vi "Framework Test2.vi"() -> ()   [LabVIEW 2017]
uses:
  Typedefs/DSF Engine Framework Configuration.ctl
  Typedefs/DSF Engine Plugin Configuration.ctl
  Typedefs/DSF Timing Info.ctl
  Typedefs/DSF Engine Plugin Thread Configuration.ctl
  Typedefs/DSF Settings Info.ctl
  Typedefs/DSF Engine Transfer Group Configuration.ctl
  Typedefs/DSF Direction.ctl
  Typedefs/DSF Engine Transfer Configuration.ctl
  Typedefs/DSF Byte Order.ctl
  Typedefs/DSF Engine Channel Configuration.ctl
  Typedefs/DSF Data Type.ctl
  Typedefs/DSF Timeout Behavior.ctl
  Classes/Framework/Framework Options.ctl
  Typedefs/DSF FIFO Options.ctl
  Classes/Thread/Thread Options.ctl
  Typedefs/DSF Plugin Options.ctl
  Typedefs/DSF Performance Options.ctl
  Classes/Framework/Data Server Options.ctl
  <vilib>/NI/Memory Manager/Classes/Pointer/Pointer.lvclass/Pointer.ctl
  <vilib>/NI/Memory Manager/Classes/Pointer/Write Bool.vi
  <vilib>/NI/Memory Manager/Classes/Pointer/Write DBL.vi
  <vilib>/NI/Memory Manager/Classes/Pointer/Read Bool.vi
  <vilib>/NI/Memory Manager/Classes/Pointer/Set Address.vi
  <vilib>/NI/Memory Manager/Classes/Pointer/Set Size.vi
  <vilib>/NI/Memory Manager/Classes/Pointer/Set Internal.vi
  <vilib>/NI/Memory Manager/Classes/Pointer/Write (No Check).vi
  <vilib>/NI/Memory Manager/Classes/Pointer/Write (No Check) Bool.vi
  <vilib>/NI/Memory Manager/Classes/Pointer/Check Move.vi
  <vilib>/NI/Memory Manager/Classes/Pointer/Check Null Pointer.vi
  <vilib>/NI/Memory Manager/Classes/Pointer/Clear (No Check).vi
  <vilib>/NI/Memory Manager/Classes/Pointer/Check Length.vi
  <vilib>/NI/Memory Manager/Classes/Pointer/Write (No Check) DBL.vi
  <vilib>/NI/Memory Manager/Classes/Pointer/Read (No Check).vi
  <vilib>/NI/Memory Manager/Classes/Pointer/Read (No Check) Bool.vi
  <vilib>/NI/Memory Manager/Classes/Pointer/Get Internal.vi
  <vilib>/NI/Memory Manager/Classes/Pointer/Errors.vi
  <vilib>/NI/Memory Manager/Classes/Pointer/Zone.vi
  <vilib>/NI/Memory Manager/Classes/Pointer/Check Count.vi
  <vilib>/NI/Memory Manager/Classes/Pointer/Check Bounds (Power of 2).vi
  <vilib>/NI/Memory Manager/Classes/Pointer/Null Pointer.vi
  <vilib>/NI/Memory Manager/Classes/Pointer/Is Null.vi
  <vilib>/NI/Memory Manager/Classes/Pointer/Check Bounds (Pointer).vi
  <vilib>/NI/Memory Manager/Classes/Pointer/Create Error.vi
  <vilib>/NI/Memory Manager/Classes/Pointer/Out of Bounds.vi
  <vilib>/NI/Memory Manager/Classes/Pointer/Check Bounds.vi
  <vilib>/NI/Memory Manager/Constants/Constants.vi
  <vilib>/NI/Memory Manager/Constants/Library Name.vi
  <vilib>/NI/Memory Manager/Classes/Pointer/Pointer Error Info.vi
  <vilib>/NI/Memory Manager/Constants/Pointer Class Name.vi
  <vilib>/NI/Memory Manager/Classes/Pointer/Write Pointer Size to Error.vi
  <vilib>/NI/Memory Manager/Classes/Pointer/Check Bounds (Buffer).vi
  <vilib>/NI/Memory Manager/Classes/Pointer/Buffer Underflow.vi
  <vilib>/NI/Memory Manager/VIs/New Error Cluster.vi
  <vilib>/NI/Memory Manager/VIs/New Error Cluster (512B).vi
  <vilib>/NI/Memory Manager/VIs/Set Error Status.vi
  <vilib>/NI/Memory Manager/VIs/Set Error Code.vi
  <vilib>/NI/Memory Manager/VIs/Set Error Source.vi
  <vilib>/NI/Memory Manager/VIs/Write String to Source.vi
  <vilib>/NI/Memory Manager/VIs/Write Numeric to Source.vi
  <vilib>/NI/Memory Manager/VIs/Write Numeric Scalar to Source (Base10 U64).vi
  <vilib>/NI/Memory Manager/Classes/Pointer/Pointer.lvclass
  Classes/Framework/Framework.lvclass
  Classes/Configuration/Configuration Session.lvclass
  DSF Core.lvlib
  Classes/Thread/Thread.lvclass
panel:
  in  "first channel":dbl
  in  "components directory":path
  in  "dsf configuration file path":path=path "C:/Users/Admin/Desktop/test.dsf"
  out "iteration":u64
  out "error out":errorcluster
  in  "framework options":T1={"FIFO Options"={"Infinite Timeouts"=FALSE}, "Thread Options"={"Show FP On Call"=TRUE, "Close FP After Call"=TRUE, "Allow Debugging"=TRUE}, "Plugin Options"={"Default Components"=TRUE}, "Performance Options"={"Measure Period"=TRUE, "Measure Rx/Tx Duration"=TRUE}, "Data Server Options"={"Enable Data Server"=TRUE, "Period"=50}} {"Data Server Options"."Period" format="%d ms"}
  in  "framework configuration":T7={"Plugins"=[{"name"="UDP", "components"=["UDP"], "cycle timing"={"priority"=100, "decimation"=1, "offset"=0}, "threads"=[{"buffer converter settings"=[], "transceiver settings"=[{"key"="Local Port", "value"="50000"}], "custom settings"=[], "processor"=-2, "priority offset"=0}, {"buffer converter settings"=[], "transceiver settings"=[{"key"="Local Port", "value"="50001"}], "custom settings"=[], "processor"=-2, "priority offset"=0}, {"buffer converter settings"=[], "transceiver settings"=[{"key"="Local Port", "value"="50002"}], "custom settings"=[], "processor"=-2, "priority offset"=0}, {"buffer converter settings"=[], "transceiver settings"=[{"key"="Local Port", "value"="50003"}], "custom settings"=[], "processor"=-2, "priority offset"=0}], "Transfer Groups"=[{"name"="Group0", "direction"=enum."Tx", "cycle timing"={"priority"=100, "decimation"=1, "offset"=0}, "thread index"=0, "settings"=[], "Transfers"=[{"name"="Transfer0", "byte order"=enum."big-endian", "settings"=[{"key"="Destination Port", "value"="60000"}, {"key"="Destination Address", "value"="localhost"}], "channels"=[{"string offset"=0, "string data type"=enum."SGL", "engine data type"=enum."DBL", "name"="Temp", "settings"=[], "units"="V"}, {"string offset"=4, "string data type"=enum."DBL", "engine data type"=enum."DBL", "name"="RPM", "settings"=[], "units"="V"}, {"string offset"=12, "string data type"=enum."Bool", "engine data type"=enum."DBL", "name"="LED", "settings"=[], "units"="V"}, {"string offset"=792, "string data type"=enum."U64", "engine data type"=enum."DBL", "name"="Count", "settings"=[], "units"="V"}]}], "timeout behavior"=enum."Increment Late Count"}], "settings"=[]}]}
  in  "stop":bool
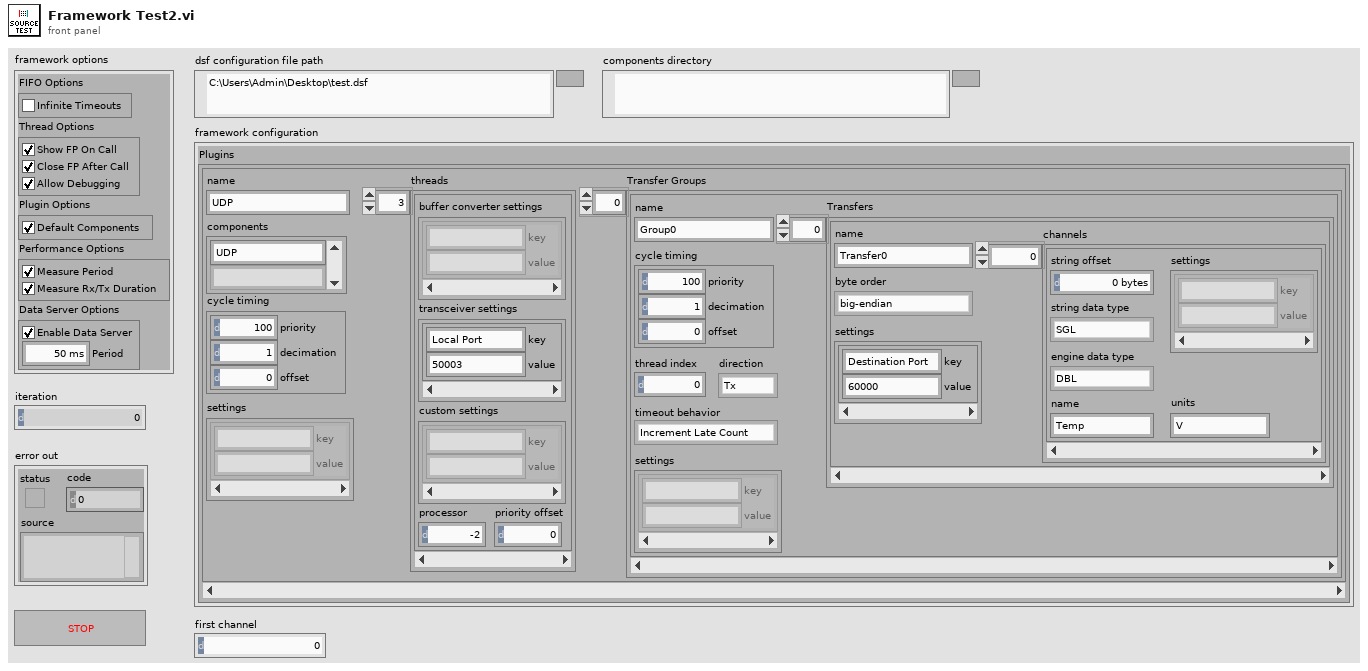
[diagram p1: front panel]
types:
  T1 = typedef "DSF Core.lvlib/Framework.lvclass/Framework Options.ctl" = cluster{"FIFO Options":T2, "Thread Options":T3, "Plugin Options":T4, "Performance Options":T5, "Data Server Options":T6}
  T2 = typedef "DSF Core.lvlib/Framework.lvclass/DSF FIFO Options.ctl" = cluster{"Infinite Timeouts":bool}
  T3 = typedef "DSF Core.lvlib/Thread.lvclass/Thread Options.ctl" = cluster{"Show FP On Call":bool, "Close FP After Call":bool, "Allow Debugging":bool}
  T4 = typedef "DSF Core.lvlib/Framework.lvclass/DSF Plugin Options.ctl" = cluster{"Default Components":bool}
  T5 = typedef "DSF Core.lvlib/DSF Performance Options.ctl" = cluster{"Measure Period":bool, "Measure Rx/Tx Duration":bool}
  T6 = typedef "DSF Core.lvlib/Framework.lvclass/Data Server Options.ctl" = cluster{"Enable Data Server":bool, "Period":u32}
  T7 = typedef "DSF Core.lvlib/DSF Engine Framework Configuration.ctl" = cluster{"Plugins":T8[]}
  T8 = typedef "DSF Core.lvlib/DSF Engine Plugin Configuration.ctl" = cluster{"name":string, "components":string[], "cycle timing":T9, "threads":T10[], "Transfer Groups":T12[], "settings":T11}
  T9 = typedef "DSF Core.lvlib/DSF Timing Info.ctl" = cluster{"priority":u64, "decimation":u64, "offset":u64}
  T10 = typedef "DSF Core.lvlib/DSF Engine Plugin Thread Configuration.ctl" = cluster{"buffer converter settings":T11, "transceiver settings":T11, "custom settings":T11, "processor":i32, "priority offset":i16}
  T11 = typedef "DSF Core.lvlib/DSF Settings Info.ctl" = cluster{"key":string, "value":string}[]
  T12 = typedef "DSF Core.lvlib/DSF Engine Transfer Group Configuration.ctl" = cluster{"name":string, "direction":T13, "cycle timing":T9, "thread index":i32, "settings":T11, "Transfers":T14[], "timeout behavior":T18}
  T13 = typedef "DSF Core.lvlib/DSF Direction.ctl" = enum8{"Tx", "Rx"}
  T14 = typedef "DSF Core.lvlib/DSF Engine Transfer Configuration.ctl" = cluster{"name":string, "byte order":T15, "settings":T11, "channels":T16[]}
  T15 = typedef "DSF Core.lvlib/DSF Byte Order.ctl" = enum8{"big-endian", "little-endian"}
  T16 = typedef "DSF Core.lvlib/DSF Engine Channel Configuration.ctl" = cluster{"string offset":u64, "string data type":T17, "engine data type":T17, "name":string, "settings":T11, "units":string}
  T17 = typedef "DSF Core.lvlib/DSF Data Type.ctl" = enum8{"Bool", "SGL", "DBL", "I8", "I16", "I32", "I64", "U8", "U16", "U32", "U64"}
  T18 = typedef "DSF Core.lvlib/DSF Timeout Behavior.ctl" = enum8{"Increment Late Count", "Throw Error"}
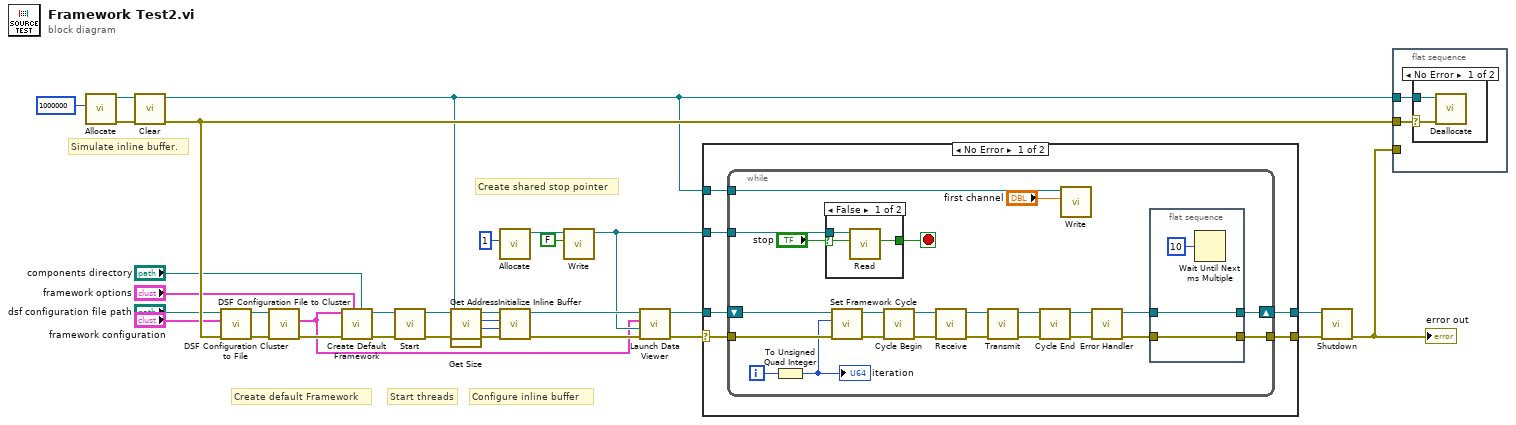
[diagram p0: block diagram]
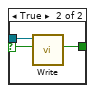
[diagram p3: hidden frame]
diagram:
  # "Create shared stop pointer"
  # "Configure inline buffer"
  # "Start threads"
  # "Create default Framework"
  # "Simulate inline buffer."
  n1 = call <vilib>:"Allocate.vi"("size"=u64 1000000) -> ("error out"=w25:errorcluster, "Pointer out"=w18:refnum<class "Pointer.lvclass">)  [unwired: 9 in]
  n2 = call <vilib>:"Clear.vi"("error in (no error)"=w25, "Pointer in"=w18) -> ("error out"=w29:errorcluster, "Pointer out"=w1:refnum<class "Pointer.lvclass">)  [unwired: 8 in]
  n3 = call "DSF Configuration Cluster to File.vi"("error in (no error)"=w29, "framework configuration"="framework configuration", "dsf configuration file path"="dsf configuration file path") -> ("error out"=w24:errorcluster, "dsf configuration file path dup"=w23:path)  [unwired: 7 in]
  n4 = call "DSF Configuration File to Cluster.vi"("error in (no error)"=w24, "dsf configuration file path"=w23) -> ("error out"=w17:errorcluster, "framework configuration out"=w6:T7)  [unwired: 7 in, 1 out]
  n5 = call "Create Default Framework.vi"("components directory (default)"="components directory", "framework options"="framework options", "error in (no error)"=w17, "framework configuration"=w6) -> ("error out"=w4:errorcluster, "Framework"=w15:refnum<class "Framework.lvclass">)  [unwired: 6 in]
  n6 = call-dynamic "Start.vi"("error in (no error)"=w4, "Framework in"=w15) -> ("error out"=w14:errorcluster, "Framework out"=w30:refnum<class "Framework.lvclass">)  [unwired: 8 in]
  n7 = call <vilib>:"Get Address.vi"("Pointer in"=w1) -> ("address"=w21:u64)  [unwired: 9 in, 1 out]
  n8 = call <vilib>:"Get Size.vi"("Pointer in"=w1) -> ("size"=w22:u64)  [unwired: 9 in, 1 out]
  n9 = call <vilib>:"Allocate.vi"("size"=u64 1) -> ("Pointer out"=w10:refnum<class "Pointer.lvclass">)  [unwired: 9 in, 1 out]
  n10 = call "Initialize Inline Buffer.vi"("error in (no error)"=w14, "size"=w22, "address"=w21, "Framework in"=w30) -> ("error out"=w12:errorcluster, "Framework out"=w13:refnum<class "Framework.lvclass">)  [unwired: 6 in]
  n11 = call-poly <vilib>:"Write.vi"("value"=FALSE, "Pointer in"=w10) -> ("Pointer out"=w9:refnum<class "Pointer.lvclass">)  [unwired: 6 in, 3 out]
  n12 = call "Launch Data Viewer.vi"("error in (no error)"=w12, "Stop Pointer"=w9, "Framework Configuration"=w6, "Framework in"=w13) -> ("error out"=w19:errorcluster, "Framework out"=w20:refnum<class "Framework.lvclass">)  [unwired: 6 in]
  n13 = case shown="No Error" w19 {
    selector: w19 -> [w35 w69]
    tunnel: [w33 w69] -> w28
    tunnel: w20 -> [w36 w70]
    tunnel: [w34 w70] -> w27
    tunnel: w9 -> [w32 _]
    tunnel: w1 -> [w31 _]
    frame No Error {
      n14 = while {
        shift-right: [w57] -> w34
        shift-left: w36 -> [w51]
        tunnel: w32 -> [w54]
        tunnel: w35 -> [w50]
        tunnel: [w56] -> w33
        tunnel: w31 -> [w38]
        i -> [w55]
        stop <- w52 stop-if-true
        n15 = To Unsigned Quad Integer(1:w55) -> (0:w49:u64)
        "iteration" <- w49
        n16 = case shown="False" "stop" {
          selector: "stop" -> [w61 w64]
          tunnel: w54 -> [w62 w65]
          tunnel: [w60 w63] -> w52
          frame False {
            n17 = call-poly <vilib>:"Read.vi"("value in"=w61, "Pointer in"=w62) -> ("value out"=w60:bool)  [unwired: 6 in, 3 out]
          }
          frame True {
            n18 = call-poly <vilib>:"Write.vi"("value"=w64, "Pointer in"=w65) -> ("value"=w63:bool)  [unwired: 6 in, 3 out]
          }
        }
        n19 = call "Set Framework Cycle.vi"("error in (no error)"=w50, "iteration"=w49, "Framework in"=w51) -> ("error out"=w47:errorcluster, "Framework out"=w48:refnum<class "Framework.lvclass">)  [unwired: 7 in]
        n20 = call "Cycle Begin.vi"("error in (no error)"=w47, "Framework in"=w48) -> ("error out"=w45:errorcluster, "Framework out"=w46:refnum<class "Framework.lvclass">)  [unwired: 8 in]
        n21 = call "Receive.vi"("error in (no error)"=w45, "Framework in"=w46) -> ("error out"=w59:errorcluster, "Framework out"=w58:refnum<class "Framework.lvclass">)  [unwired: 8 in]
        n22 = call "Transmit.vi"("error in (no error)"=w59, "Framework in"=w58) -> ("error out"=w43:errorcluster, "Framework out"=w44:refnum<class "Framework.lvclass">)  [unwired: 8 in]
        n23 = call "Cycle End.vi"("error in (no error)"=w43, "Framework in"=w44) -> ("error out"=w41:errorcluster, "Framework out"=w42:refnum<class "Framework.lvclass">)  [unwired: 8 in]
        n24 = call-poly <vilib>:"Write.vi"("value"="first channel", "Pointer in"=w38) -> ()  [unwired: 6 in, 4 out]
        n25 = call "Error Handler.vi"("error in (no error)"=w41, "Framework in"=w42) -> ("error out"=w39:errorcluster, "Framework out"=w40:refnum<class "Framework.lvclass">)  [unwired: 8 in]
        n26 = flat-sequence {
          tunnel: w40 -> [w67]
          tunnel: w39 -> [w66]
          tunnel: [w67] -> w57
          tunnel: [w66] -> w56
          frame #0 {
            n27 = Wait Until Next ms Multiple(millisecond multiple=u32 10 ("milliseconds to wait")) -> ()  [unwired: 1 out]
          }
        }
      }
    }
    frame Error {
    }
  }
  n28 = call-dynamic "Shutdown.vi"("error in (no error)"=w28, "Framework in"=w27) -> ("error out"=w2:errorcluster)  [unwired: 8 in, 1 out]
  "error out" <- w2
  n29 = flat-sequence {
    tunnel: w1 -> [w72]
    tunnel: w2 -> [_]
    tunnel: w29 -> [w71]
    frame #0 {
      n30 = case shown="No Error" w71 {
        selector: w71 -> [w73 _]
        tunnel: w72 -> [w74 _]
        frame No Error {
          n31 = call <vilib>:"Deallocate.vi"("error in (no error)"=w73, "Pointer"=w74) -> ()  [unwired: 8 in, 2 out]
        }
        frame Error {
        }
      }
    }
  }
